vi "23384_Davis_Poku_Amankwa_Amankwa.DavisPoku.MNE1201.1.8_348252_1910191105.vi"() -> ()   [LabVIEW 2018]
panel:
  out "A and B":bool
  in  "B":bool
  in  "A":bool
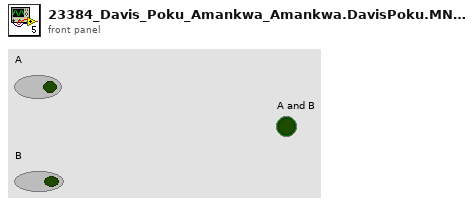
[diagram p1: front panel]
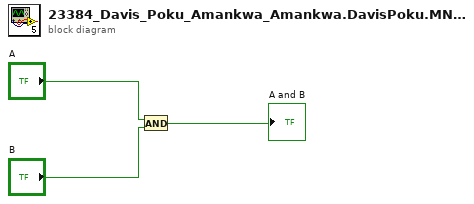
[diagram p0: block diagram]
diagram:
  n1 = And(x="A", y="B") -> (x .and. y?=→"A and B":bool)
